vi "ecuacion caracteristica LDR(SubVI).vi"(8 "Error In":errorcluster, 11 "LDR":dbl) -> (0 "Error Out":errorcluster, 3 "Miles de lumenes":dbl)   [LabVIEW 2013]
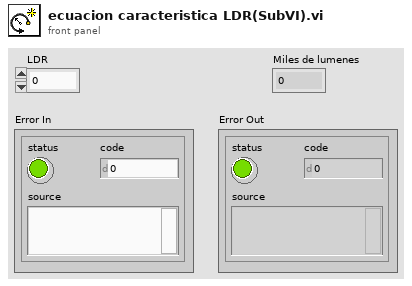
[diagram p1: front panel]
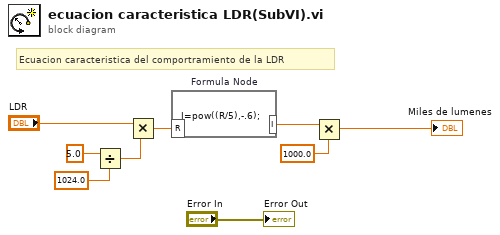
[diagram p0: block diagram]
diagram:
  # "Ecuacion caracteristica del comportramiento de la LDR"
  n1 = Divide(x=5.0, y=1024.0) -> (x/y=w5:dbl)
  n2 = Multiply(x="LDR", y=w5) -> (x*y=w6:dbl)
  n3 = formula code="I=pow((R/5),-.6);"("R"=w6) -> ("I"=w7:dbl)
  n4 = Multiply(x=w7, y=1000.0) -> (x*y=→"Miles de lumenes":dbl)
  "Error Out" <- "Error In"
